vi "CRYAutoProtect All.vi"(11 "Delete?":bool=TRUE) -> (1 "AutoProtect?":bool=TRUE, 2 "AutoProtected Array Out":i32[](array[numeric]))   [LabVIEW 2013]
panel:
  # "Unprotect All Data(Curves, Values,Results, Waveforms)"
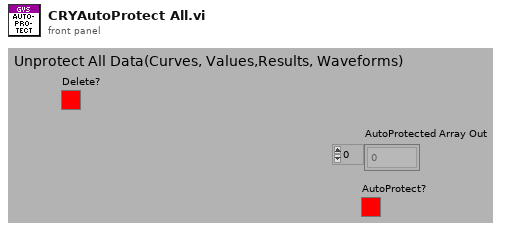
[diagram p1: front panel]
types:
  T1 = typedef "CRYData Cluster.ctl" = cluster{"Name":string, "Curve":cluster{"x":dbl, "y":dbl, "z":dbl}[], "X data":u16, "Y data":u16, "Z data":u16, "X axis":u16, "Y axis":u16, "Z axis":u16, "X unit":string, "Y unit":string, "Z unit":string, "X dB ref":dbl, "Y dB ref":dbl, "Z dB ref":dbl, "single val":bool, "protected":bool, "display X":bool, "display Y":bool, "display Z":bool, "Test Info":string, "Step No.":i32, "Plot Settings":cluster{"Color":u32, "Interpolation":u8, "Point Style":u8, "Line Style":u8, "Point Color":u32, "Line Width":u8, "Bar Plot Style":u8, "Fill To":i16}, "AutoProtect":bool}
  T2 = typedef "CRYWaveform Cluster.ctl" = cluster{"Waveform":cluster{"X0":dbl, "dX":dbl, "Y":sgl[]}, "X data":u16, "Y data":u16, "Y axis":u16, "X unit":string, "Y unit":string, "Y dB ref":dbl, "display Y":bool, "display X":bool, "Overload?":bool, "Test Info":string, "Step No.":i32, "Name":string, "protected":bool, "Sqc history":string[], "Signal Channel ID":i32, "Plot Settings":cluster{"Color":u32, "Interpolation":u8, "Point Style":u8, "Line Style":u8, "Point Color":u32, "Line Width":u8, "Bar Plot Style":u8, "Fill To":i16}, "AutoProtect":bool}
  T3 = typedef "CRYResult Cluster.ctl" = cluster{"Name":string, "Margin":dbl, "unit":string, "Verdict":bool, "Limit":string, "Max/Min":string, "protected":bool, "Step No.":i32, "Test Info":string, "AutoProtect":bool}
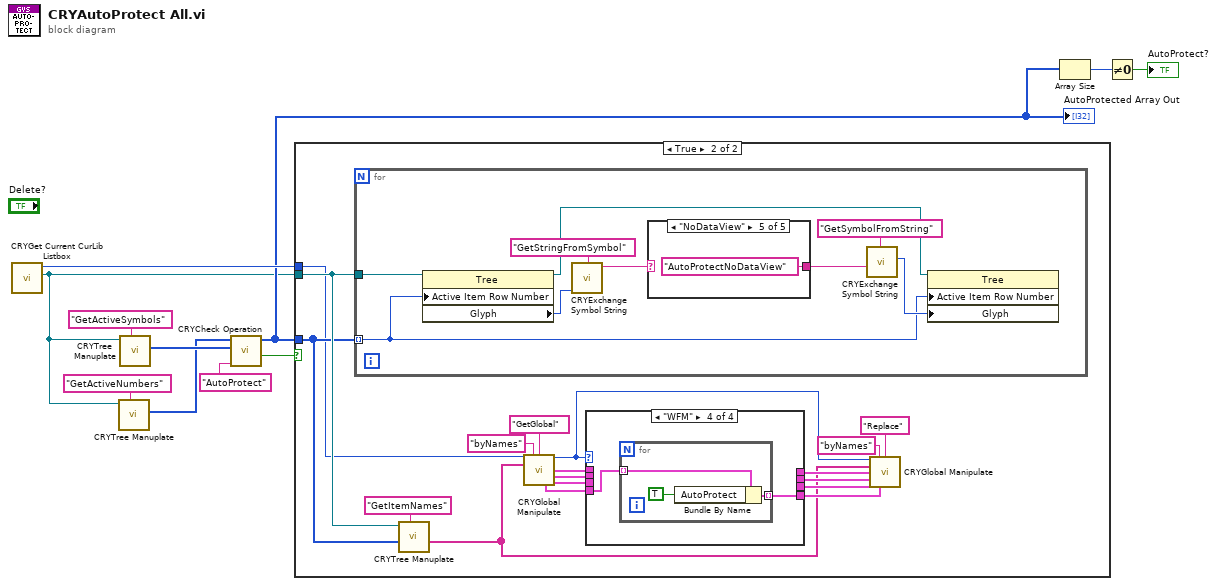
[diagram p0: block diagram]
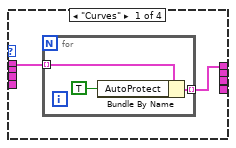
[diagram p3: hidden frame]
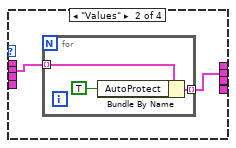
[diagram p4: hidden frame]
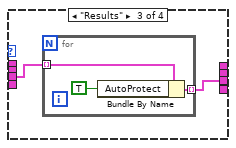
[diagram p5: hidden frame]
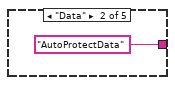
[diagram p7: hidden frame]
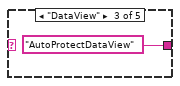
[diagram p8: hidden frame]
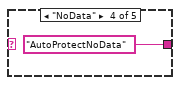
[diagram p9: hidden frame]
diagram:
  n1 = call "CRYGet Current CurLib Listbox.vi"() -> ("CurLib Tree"=w1:refnum<vi>, "Type"=w8:enum16{"Curves", "Values", "Results", "WFM"})  [unwired: 9 in, 1 out]
  n2 = call "CRYTree Manuplate.vi"("sAction"="GetActiveNumbers", "Tree in"=w1) -> ("nData Out"=w2:i32[])  [unwired: 6 in, 3 out]
  n3 = call "CRYTree Manuplate.vi"("sAction"="GetActiveSymbols", "Tree in"=w1) -> ("nData Out"=w3:i32[])  [unwired: 6 in, 3 out]
  n4 = call "CRYCheck Operation.vi"("Operation"="AutoProtect", "Item Symbols In"=w3, "Index Array In"=w2) -> ("Operation ?"=w6:bool, "Array Out"=w7:i32[])  [unwired: 6 in, 1 out]
  "AutoProtected Array Out" <- w7
  n5 = case shown="True" w6 {
    tunnel: w7 -> [_ w15]
    tunnel: w8 -> [_ w13]
    tunnel: w1 -> [_ w16]
    frame False {
    }
    frame True {
      n6 = for {
        tunnel: w15 -> [w50] mode=indexing
        tunnel: w16 -> [w51]
        n7 = property on="Property Node" class="Tree"(reference=w51, "Active Item Row Number"=w50) -> (reference out=w52:refnum<vi>, "Glyph"=w57:i32)  [unwired: 1 in, 1 out]
        n8 = call "CRYExchange Symbol String.vi"("nData"=w57, "sAction"="GetStringFromSymbol") -> ("sData out"=w54:string)  [unwired: 8 in, 1 out]
        n9 = case shown="\"NoDataView\"" w54 {
          selector: w54 -> [w59 _ _ _ _]
          tunnel: [w59 "AutoProtectData" ("sAction") "AutoProtectDataView" ("sAction") "AutoProtectNoData" ("sAction") "AutoProtectNoDataView" ("sAction")] -> w53
          frame Default {
          }
          frame "Data" {
          }
          frame "DataView" {
          }
          frame "NoData" {
          }
          frame "NoDataView" {
          }
        }
        n10 = call "CRYExchange Symbol String.vi"("sData"=w53, "sAction"="GetSymbolFromString") -> ("nData out"=w55:i32)  [unwired: 8 in, 1 out]
        n11 = property on="Property Node" class="Tree"(reference=w52, "Active Item Row Number"=w50, "Glyph"=w55) -> ()  [unwired: 1 in, 2 out]
      }
      n12 = call "CRYTree Manuplate.vi"("sAction"="GetItemNames", "nData"=w15, "Tree in"=w16) -> ("sData Out"=w14:string[])  [unwired: 5 in, 3 out]
      n13 = call "CRYGlobal Manipulate.vi"("Type"=w13, "sOption"="byNames", "sAction"="GetGlobal", "sData"=w14) -> ("Type out"=w24:enum16{"Curves", "Values", "Results", "WFM"}, "Curves Out"=w29:T1[], "Values Out"=w23:T1[], "WFM Out"=w21:T2[], "Results Out"=w22:T3[])  [unwired: 5 in, 2 out]
      n14 = case shown="\"WFM\"" w24 {
        tunnel: w29 -> [w31 _ _ _]
        tunnel: [w30 _ _ _] -> w25
        tunnel: w23 -> [_ w36 _ _]
        tunnel: w22 -> [_ _ w41 _]
        tunnel: w21 -> [_ _ _ w46]
        tunnel: [_ w35 _ _] -> w20
        tunnel: [_ _ w40 _] -> w19
        tunnel: [_ _ _ w45] -> w18
        frame "Curves" {
          n15 = for {
            tunnel: w31 -> [w32] mode=indexing
            tunnel: [w33] -> w30 mode=indexing
            n16 = Bundle By Name(cluster=w32, "AutoProtect"=TRUE ("protected")) -> (w33:T1)
          }
        }
        frame "Values" {
          n17 = for {
            tunnel: w36 -> [w37] mode=indexing
            tunnel: [w38] -> w35 mode=indexing
            n18 = Bundle By Name(cluster=w37, "AutoProtect"=TRUE ("protected")) -> (w38:T1)
          }
        }
        frame "Results" {
          n19 = for {
            tunnel: w41 -> [w42] mode=indexing
            tunnel: [w43] -> w40 mode=indexing
            n20 = Bundle By Name(cluster=w42, "AutoProtect"=TRUE ("protected")) -> (w43:T3)
          }
        }
        frame "WFM" {
          n21 = for {
            tunnel: w46 -> [w47] mode=indexing
            tunnel: [w48] -> w45 mode=indexing
            n22 = Bundle By Name(cluster=w47, "AutoProtect"=TRUE ("protected")) -> (w48:T2)
          }
        }
      }
      n23 = call "CRYGlobal Manipulate.vi"("Type"=w24, "sOption"="byNames", "sAction"="Replace", "sData"=w14, "Curves"=w25, "Values"=w20, "Results"=w19, "WFM"=w18) -> ()  [unwired: 1 in, 7 out]
    }
  }
  n24 = Array Size(array=w7) -> (size(s)=w11:i32)
  n25 = Not Equal To 0?(x=w11) -> (x != 0?=→"AutoProtect?":bool)
